vi "Untitled 1.vi"() -> ()   [LabVIEW 2021]
uses:
  <vilib>/Instr/_visa.llb/VISA Configure Serial Port (Instr).vi
panel:
  in  "Baud Rate:":u32=9600
  in  "stop":bool
  in  "Port:":refnum<visa-resource-name>
  out "Nem Yüksek":bool
  out "Nem Düþük":bool
  out "Pompa":bool
  out "% Nem":dbl(slide) scale=0.0..100.0 scale format="%_1p"
  out "read buffer":string
  # "Seri Haberleþme\nAyarlarý"
  # "Otomatik Çiçek Sulama Sistemi"
  # "% Nem"
  # "Pompa Çalýþýyor"
  # "Nem Seviyesi Çok Düþük (<%25)"
  # "Nem Seviyesi Çok Yüksek (>%75)"
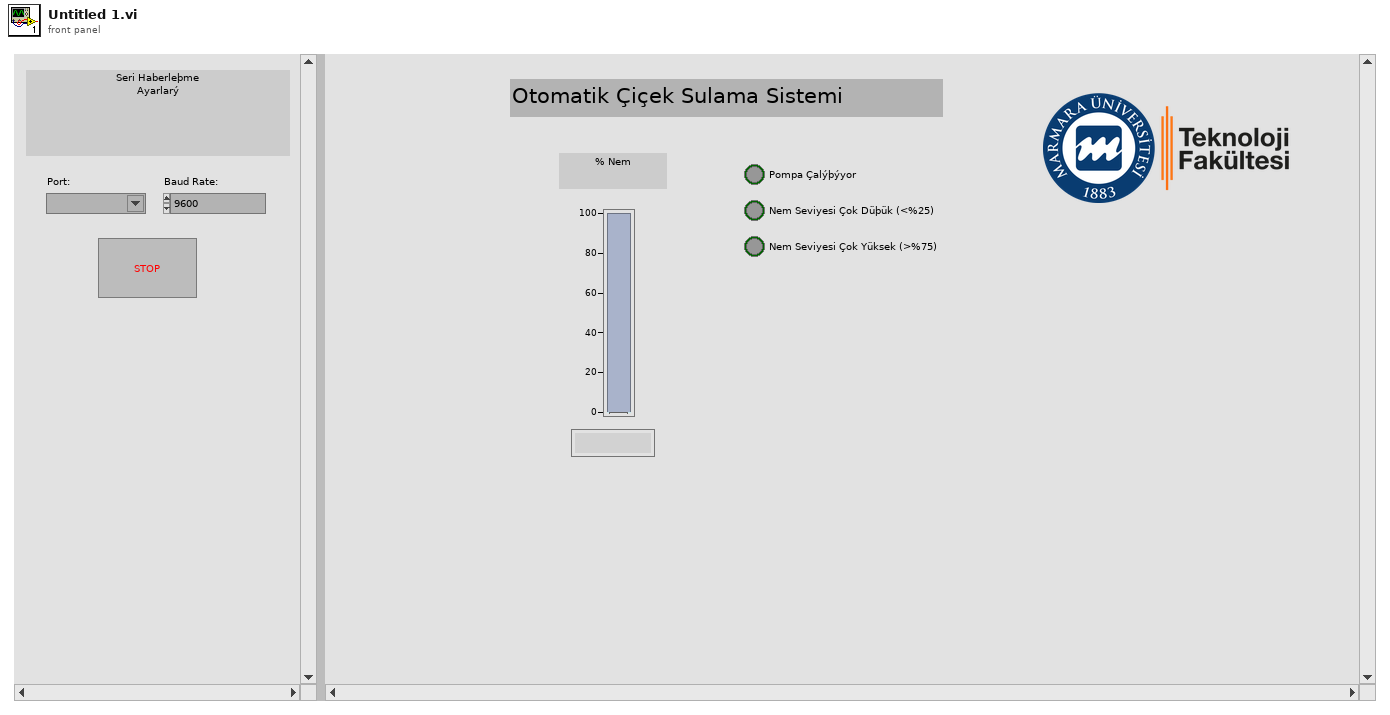
[diagram p1: front panel]
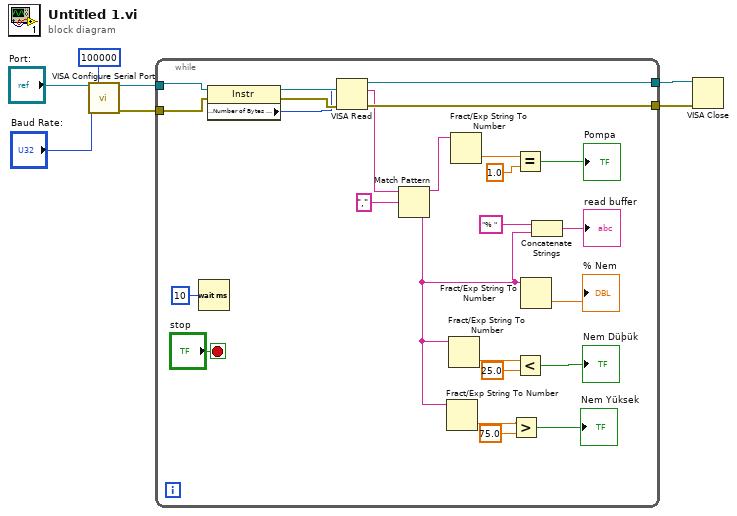
[diagram p0: block diagram]
diagram:
  n1 = call-poly "VISA Configure Serial Port"("VISA resource name"="Port:", "timeout (10sec)"=u32 100000, "baud rate (9600)"="Baud Rate:") -> ("VISA resource name out"=w6:refnum<visa-resource-name>, "error out"=w5:errorcluster)  [unwired: 11 in]
  n2 = while {
    tunnel: w6 -> [w25]
    tunnel: w5 -> [w24]
    tunnel: [w28] -> w4
    tunnel: [w27] -> w3
    stop <- "stop" stop-if-true
    n3 = Wait (ms)(milliseconds to wait=u32 10) -> ()  [unwired: 1 out]
    n4 = property class="Instr"(reference=w25, error in=w24) -> (reference out=w32:refnum<visa-resource-name>, error out=w31:errorcluster, "Serial Settings:Number of Bytes at Serial Port"=w30:u32)
    n5 = VISA Read(VISA resource name=w32, byte count=w30, error in (no error)=w31) -> (VISA resource name out=w28:refnum<visa-resource-name>, read buffer=w20:string, error out=w27:errorcluster)  [unwired: 1 out]
    n6 = Match Pattern(string=w20, regular expression=",") -> (before substring=w16:string, after substring=w8:string)  [unwired: 1 in, 2 out]
    n7 = Fract/Exp String To Number(string=w8) -> (number=w10:dbl)  [unwired: 3 in, 1 out]
    n8 = Fract/Exp String To Number(string=w8) -> (number=w14:dbl)  [unwired: 3 in, 1 out]
    n9 = Fract/Exp String To Number(string=w16) -> (number=w15:dbl)  [unwired: 3 in, 1 out]
    n10 = Greater?(x=w10, y=75.0) -> (0:→"Nem Yüksek":bool)
    n11 = Equal?(x=w15, y=1.0) -> (x = y?=→"Pompa":bool)
    n12 = Less?(x=w14, y=25.0) -> (x < y?=→"Nem Düþük":bool)
    n13 = Fract/Exp String To Number(string=w8) -> (number=→"% Nem":dbl)  [unwired: 3 in, 1 out]
    n14 = Concatenate Strings("% " ("string"), w8) -> (→"read buffer":string)
  }
  n15 = VISA Close(VISA resource name=w4, error in (no error)=w3) -> ()  [unwired: 1 out]
